vi "Cents2DollarString.vi"(9 "Numeric":dbl format="%#_13g") -> (0 "Dollar String Out":string)   [LabVIEW 2014]
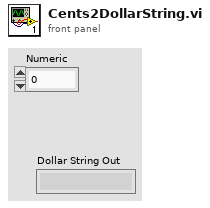
[diagram p1: front panel]
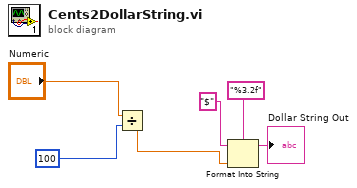
[diagram p0: block diagram]
diagram:
  n1 = Divide(x="Numeric", y=100) -> (x/y=w3:dbl)
  n2 = Format Into String(format string="%3.2f", initial string="$", w3) -> (resulting string=→"Dollar String Out":string)  [unwired: 1 in, 1 out]
